vi "radian_conversion.vi"(10 "input":dbl) -> (2 "output":dbl)   [LabVIEW 2020]
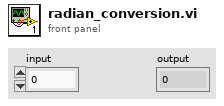
[diagram p1: front panel]
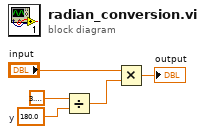
[diagram p0: block diagram]
diagram:
  w4 = 180.0  # y
  n1 = Divide(x=3.141592653589793, y=w4) -> (x/y=w5:dbl)
  n2 = Multiply(x="input", y=w5) -> (x*y=→"output":dbl)
